vi "Choreo_ByteBuffer_encode_ByteI8.vi"(9 "Int8_Value":i8, 11 "RawData In":u8[](array[numeric])) -> (3 "RawData Out":u8[](array[numeric]))   [LabVIEW 2019, in "ChoreoLib.lvlib"]
doc: "Encode (or append) an unsigned byte at the end of an array of bytes. No conversion is actually done, the memory is just copied to the end of the array.\n\nInputs\n - RawData In -- Array of bytes to be appended to..\n - Int8_Value -- Byte in the form of an INT 8 value.\n\nOutputs\n - RawData Out -- Array of bytes containing the appended value."
uses:
  ChoreoLib.lvlib
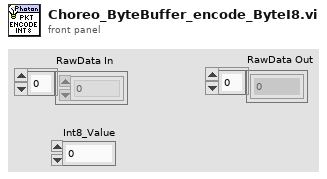
[diagram p1: front panel]
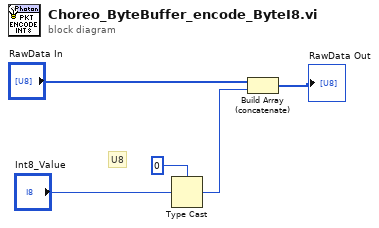
[diagram p0: block diagram]
diagram:
  # "U8"
  n1 = Type Cast(type=u8 0, x="Int8_Value") -> (*(type *) &x=w2:u8)
  n2 = Build Array (concatenate)("RawData In", w2) -> (→"RawData Out":u8[])
